vi "0520_Controle_servo_braço.vi"() -> ()   [LabVIEW 2017]
uses:
  <vilib>/Utility/error.llb/Error Cluster From Error Code.vi
  <vilib>/myRIO/Common/Instrument Driver Framework/myRIO v1.0/PWM/vis/myRIO v1.0 Write PWM.vi
  <vilib>/myRIO/Instrument Drivers/Onboard IO/PWM/PWM.lvlib
panel:
  in  "Numeric":dbl
  in  "Record Button":bool
  in  "Play Button":bool
  in  "Array":dbl[][](array[numeric])
  in  "Comprimento de pulso R7":dbl(knob)=1.5 step=0.05 scale=0.25..0.125
  out "error out 7":errorcluster
  out "error out 6":errorcluster
  out "error out 5":errorcluster
  out "error out 4":errorcluster
  out "error out 3":errorcluster
  in  "error in (no error) 7":errorcluster
  in  "error in (no error) 6":errorcluster
  in  "error in (no error) 5":errorcluster
  in  "error in (no error) 4":errorcluster
  in  "error in (no error) 3":errorcluster
  in  "Comprimento de pulso R6":dbl(knob)=90.0 min=90.0 max=300.0 step=3.0 scale=90.0..300.0
  in  "Comprimento de pulso R5":dbl(knob)=0.125 min=0.0 max=180.0 step=3.0 scale=0.0..180.0
  in  "Comprimento de pulso R4":dbl(knob) min=-180.0 max=0.0 step=3.0
  in  "Comprimento de pulso R3":dbl(knob)=0.125 min=0.025 max=0.125 step=0.001 scale=0.025..0.125
  in  "Comprimento de pulso R2":dbl(knob)=0.125 min=-90.0 max=90.0 step=1.0 scale=-90.0..90.0
  out "error out 2":errorcluster
  in  "error in (no error) 2":errorcluster
  out "error out":errorcluster
  in  "error in (no error)":errorcluster
  in  "Comprimento de pulso R1":dbl(knob)=0.125 min=0.025 max=0.125 step=0.001 scale=0.025..0.125
  in  "Stop Button":bool
  # "Range: 0,025 - 0,125\n\n3° = 0,00125\n\nLink 1 - (0,00125/3)x + 0,1\n0,125 -> 60°\n0,1 -> 0°\n0,0625 -> -90\n0,025 -> -180°\n\nLink 2 - -(0,00125/3)x + 0,1\n0,025 -> 180°\n0,0625 -> 90°\n0,1 -> 0°\n0,125 -> -60°\n\nLink 3 - (0,00125/3)x - 0,0125\n0,125 -> 300°\n0,105 -> 270° \n0,63 -> 180°\n0,025 -> 90°\n\n9° = 0,05\n\nLink 5 - (0,005/9)x + 0,075\n0,125 -> 90°\n0,075 -> 0°\n0,025 ->-90°"
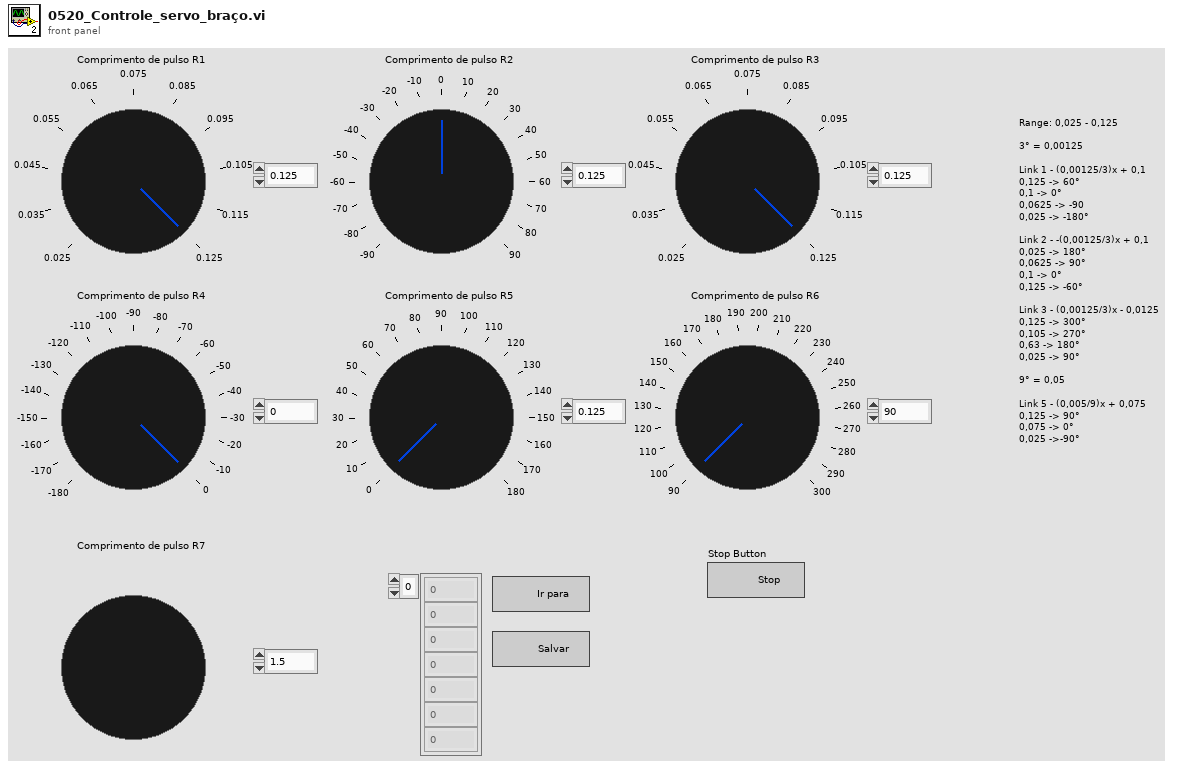
[diagram p1: front panel]
types:
  T1 = typedef "PWM.lvlib/PWM Reference.ctl" = cluster{"myRIO Reference":T2, "PWM Channels Enum":T6, "PWM Configuration":T7}
  T2 = typedef "myRIO Generic Hardware Reference.ctl" = cluster{"myRIO Model":T3, "myRIO Hardware Reference":T4}
  T3 = typedef "Hardware Version Enum.ctl" = enum16{"Unknown", "myRIO-1900", "myRIO-1950", "roboRIO", "NI ELVIS RIO CM"}
  T4 = typedef "myRIO v1.0 Reference.ctl" = cluster{"Generic FPGA Reference":T5, "Allow multiple opens":bool}
  T5 = typedef "Generic FPGA Reference.ctl" = refnum<k20>
  T6 = typedef "PWM Channels Enum.ctl" = enum16{"Not Connected", "C/PWM0", "C/PWM1", "A/PWM0", "A/PWM1", "A/PWM2", "B/PWM0", "B/PWM1", "B/PWM2", "PWM/PWM0", "PWM/PWM1", "PWM/PWM2", "PWM/PWM3", "PWM/PWM4", "PWM/PWM5", "PWM/PWM6", "PWM/PWM7", "PWM/PWM8", "PWM/PWM9"}
  T7 = typedef "PWM.lvlib/PWM Configuration.ctl" = cluster{"Frequency":dbl, "Duty Cycle":dbl}
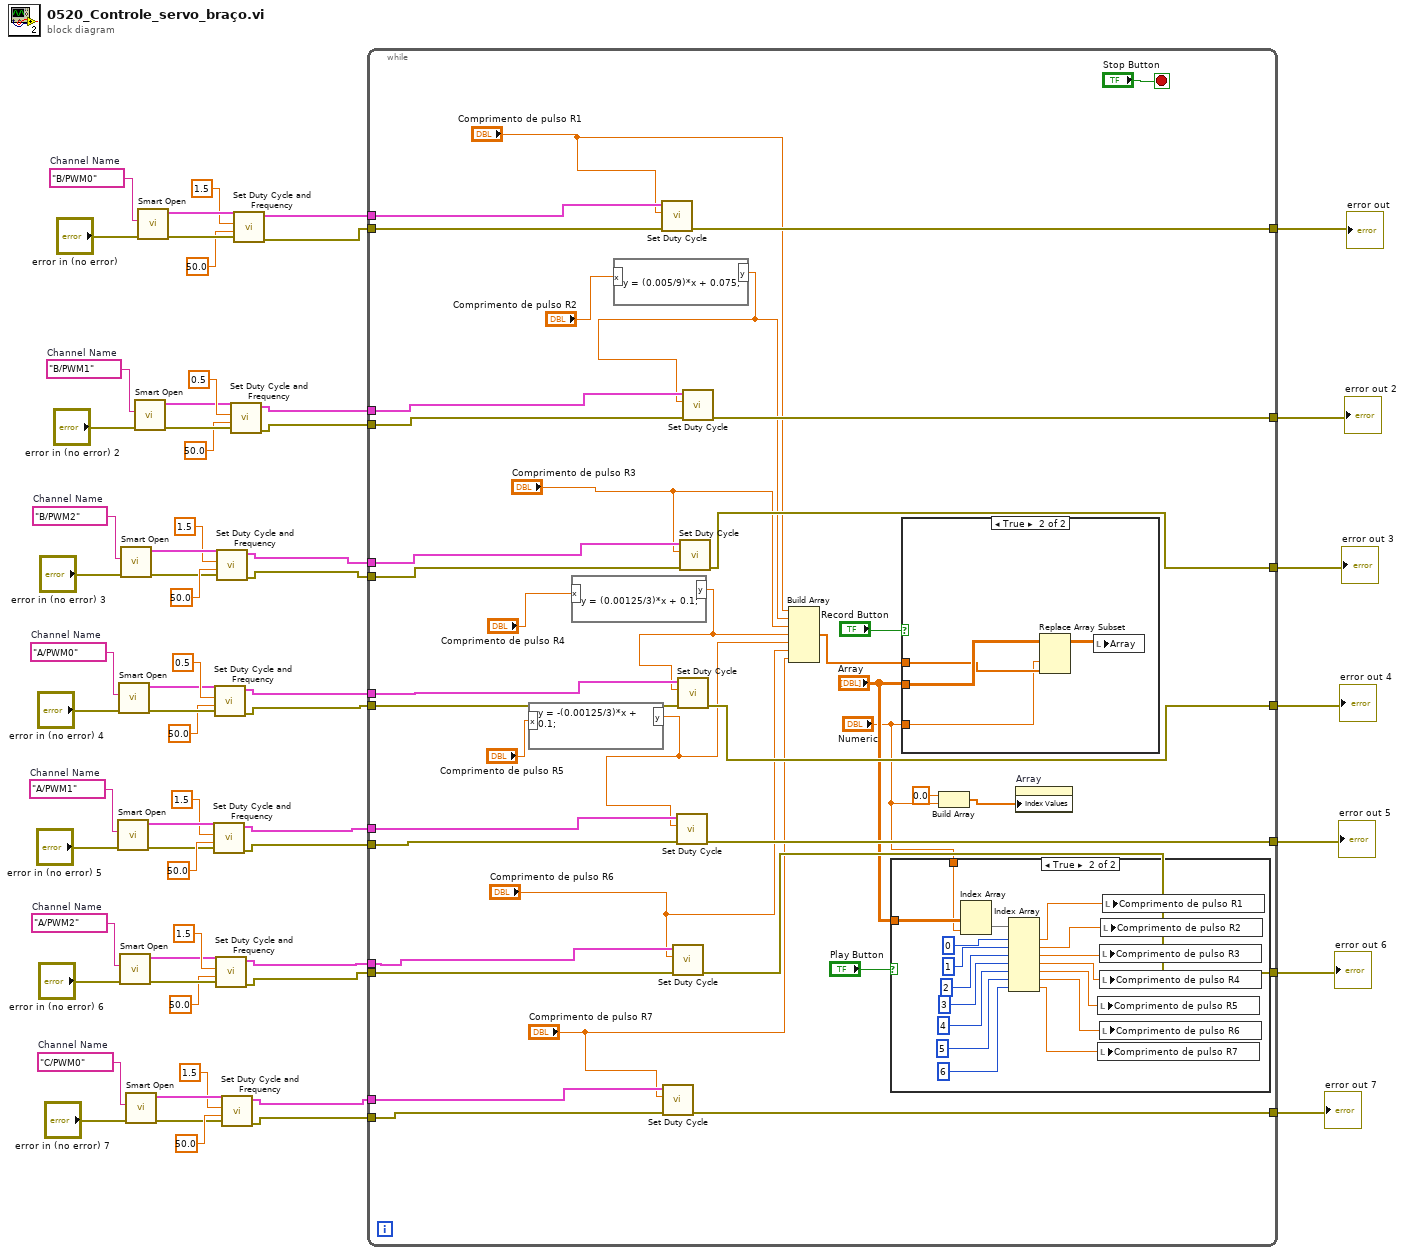
[diagram p0: block diagram]
diagram:
  w19 = tag "C/PWM0"  # Channel Name
  w24 = tag "A/PWM2"  # Channel Name
  w31 = tag "A/PWM1"  # Channel Name
  w36 = tag "A/PWM0"  # Channel Name
  w43 = tag "B/PWM2"  # Channel Name
  w52 = tag "B/PWM1"  # Channel Name
  w62 = tag "B/PWM0"  # Channel Name
  n1 = call <vilib>:"Smart Open.vi"("error in (no error)"="error in (no error) 5", "Channel Name"=w31) -> ("error out"=w30:errorcluster, "PWM Ref Out"=w29:T1)  [unwired: 8 in]
  n2 = call <vilib>:"Smart Open.vi"("error in (no error)"="error in (no error) 4", "Channel Name"=w36) -> ("error out"=w37:errorcluster, "PWM Ref Out"=w38:T1)  [unwired: 8 in]
  n3 = call <vilib>:"Smart Open.vi"("error in (no error)"="error in (no error) 6", "Channel Name"=w24) -> ("error out"=w25:errorcluster, "PWM Ref Out"=w26:T1)  [unwired: 8 in]
  n4 = call <vilib>:"Smart Open.vi"("error in (no error)"="error in (no error) 3", "Channel Name"=w43) -> ("error out"=w42:errorcluster, "PWM Ref Out"=w41:T1)  [unwired: 8 in]
  n5 = call <vilib>:"Smart Open.vi"("error in (no error)"="error in (no error) 7", "Channel Name"=w19) -> ("error out"=w18:errorcluster, "PWM Ref Out"=w17:T1)  [unwired: 8 in]
  n6 = call <vilib>:"Smart Open.vi"("error in (no error)"="error in (no error) 2", "Channel Name"=w52) -> ("error out"=w53:errorcluster, "PWM Ref Out"=w54:T1)  [unwired: 8 in]
  n7 = call <vilib>:"Smart Open.vi"("error in (no error)"="error in (no error)", "Channel Name"=w62) -> ("error out"=w61:errorcluster, "PWM Ref Out"=w60:T1)  [unwired: 8 in]
  n8 = call <vilib>:"Set Duty Cycle and Frequency.vi"("error in (no error)"=w30, "Frequency [Hz]"=50.0, "Duty Cycle"=1.5, "PWM Ref In"=w29) -> ("error out"=w6:errorcluster, "PWM Ref Out"=w5:T1)  [unwired: 5 in]
  n9 = call <vilib>:"Set Duty Cycle and Frequency.vi"("error in (no error)"=w37, "Frequency [Hz]"=50.0, "Duty Cycle"=0.5, "PWM Ref In"=w38) -> ("error out"=w4:errorcluster, "PWM Ref Out"=w3:T1)  [unwired: 5 in]
  n10 = call <vilib>:"Set Duty Cycle and Frequency.vi"("error in (no error)"=w25, "Frequency [Hz]"=50.0, "Duty Cycle"=1.5, "PWM Ref In"=w26) -> ("error out"=w8:errorcluster, "PWM Ref Out"=w7:T1)  [unwired: 5 in]
  n11 = call <vilib>:"Set Duty Cycle and Frequency.vi"("error in (no error)"=w42, "Frequency [Hz]"=50.0, "Duty Cycle"=1.5, "PWM Ref In"=w41) -> ("error out"=w2:errorcluster, "PWM Ref Out"=w1:T1)  [unwired: 5 in]
  n12 = call <vilib>:"Set Duty Cycle and Frequency.vi"("error in (no error)"=w18, "Frequency [Hz]"=50.0, "Duty Cycle"=1.5, "PWM Ref In"=w17) -> ("error out"=w9:errorcluster, "PWM Ref Out"=w10:T1)  [unwired: 5 in]
  n13 = call <vilib>:"Set Duty Cycle and Frequency.vi"("error in (no error)"=w53, "Frequency [Hz]"=50.0, "Duty Cycle"=0.5, "PWM Ref In"=w54) -> ("error out"=w49:errorcluster, "PWM Ref Out"=w50:T1)  [unwired: 5 in]
  n14 = call <vilib>:"Set Duty Cycle and Frequency.vi"("error in (no error)"=w61, "Frequency [Hz]"=50.0, "Duty Cycle"=1.5, "PWM Ref In"=w60) -> ("error out"=w58:errorcluster, "PWM Ref Out"=w59:T1)  [unwired: 5 in]
  n15 = while {
    tunnel: w59 -> [w101]
    tunnel: w58 -> [w100]
    tunnel: [w99] -> w57
    tunnel: w50 -> [w98]
    tunnel: w49 -> [w97]
    tunnel: [w96] -> w48
    tunnel: [w95] -> w15
    tunnel: [w94] -> w14
    tunnel: [w93] -> w13
    tunnel: [w92] -> w12
    tunnel: [w91] -> w11
    tunnel: w10 -> [w90]
    tunnel: w9 -> [w89]
    tunnel: w8 -> [w88]
    tunnel: w7 -> [w87]
    tunnel: w6 -> [w86]
    tunnel: w5 -> [w85]
    tunnel: w4 -> [w84]
    tunnel: w3 -> [w83]
    tunnel: w2 -> [w82]
    tunnel: w1 -> [w81]
    stop <- "Stop Button" stop-if-true
    n16 = formula code="y = -(0.00125/3)*x + 0.1;"("x"="Comprimento de pulso R5") -> ("y"=w68:dbl)
    n17 = formula code="y = (0.00125/3)*x + 0.1;"("x"="Comprimento de pulso R4") -> ("y"=w69:dbl)
    n18 = formula code="y = (0.005/9)*x + 0.075;"("x"="Comprimento de pulso R2") -> ("y"=w65:dbl)
    n19 = call <vilib>:"Set Duty Cycle.vi"("error in (no error)"=w100, "Duty Cycle"="Comprimento de pulso R1", "PWM Ref In"=w101) -> ("error out"=w99:errorcluster)  [unwired: 6 in, 1 out]
    n20 = call <vilib>:"Set Duty Cycle.vi"("error in (no error)"=w89, "Duty Cycle"="Comprimento de pulso R7", "PWM Ref In"=w90) -> ("error out"=w91:errorcluster)  [unwired: 6 in, 1 out]
    n21 = call <vilib>:"Set Duty Cycle.vi"("error in (no error)"=w88, "Duty Cycle"="Comprimento de pulso R6", "PWM Ref In"=w87) -> ("error out"=w92:errorcluster)  [unwired: 6 in, 1 out]
    n22 = call <vilib>:"Set Duty Cycle.vi"("error in (no error)"=w86, "Duty Cycle"=w68, "PWM Ref In"=w85) -> ("error out"=w93:errorcluster)  [unwired: 6 in, 1 out]
    n23 = call <vilib>:"Set Duty Cycle.vi"("error in (no error)"=w84, "Duty Cycle"=w69, "PWM Ref In"=w83) -> ("error out"=w94:errorcluster)  [unwired: 6 in, 1 out]
    n24 = call <vilib>:"Set Duty Cycle.vi"("error in (no error)"=w82, "Duty Cycle"="Comprimento de pulso R3", "PWM Ref In"=w81) -> ("error out"=w95:errorcluster)  [unwired: 6 in, 1 out]
    n25 = call <vilib>:"Set Duty Cycle.vi"("error in (no error)"=w97, "Duty Cycle"=w65, "PWM Ref In"=w98) -> ("error out"=w96:errorcluster)  [unwired: 6 in, 1 out]
    n26 = Build Array("Comprimento de pulso R1", w65, "Comprimento de pulso R3", w69, w68, "Comprimento de pulso R6", "Comprimento de pulso R7") -> (w79:dbl[])
    n27 = case shown="True" "Play Button" {
      tunnel: "Array" -> [_ w119]
      tunnel: "Numeric" -> [_ w118]
      frame False {
      }
      frame True {
        n28 = Index Array(array=w119, index (col)=w118) -> (element=w117:dbl[])  [unwired: 1 in]
        n29 = Index Array(array=w117, index #1=0 ("index"), index #2=1 ("index"), index #3=2 ("index"), index #4=3 ("index"), index #5=4 ("index"), index #6=5 ("index"), index #7=6 ("index")) -> (element #1=w109:dbl, element #2=w108:dbl, element #3=w107:dbl, element #4=w106:dbl, element #5=w105:dbl, element #6=w104:dbl, element #7=w103:dbl)
        n30 = local write "Comprimento de pulso R5"(w105) -> ()
        n31 = local write "Comprimento de pulso R7"(w103) -> ()
        n32 = local write "Comprimento de pulso R3"(w107) -> ()
        n33 = local write "Comprimento de pulso R4"(w106) -> ()
        n34 = local write "Comprimento de pulso R6"(w104) -> ()
        n35 = local write "Comprimento de pulso R2"(w108) -> ()
        n36 = local write "Comprimento de pulso R1"(w109) -> ()
      }
    }
    n37 = case shown="True" "Record Button" {
      tunnel: "Array" -> [_ w123]
      tunnel: w79 -> [_ w121]
      tunnel: "Numeric" -> [_ w120]
      frame False {
      }
      frame True {
        n38 = Replace Array Subset(array=w123, new element=w121, index (col)=w120) -> (w122:dbl[][])  [unwired: 1 in]
        n39 = local write "Array"(w122) -> ()
      }
    }
    n40 = Build Array(0.0 ("element"), "Numeric") -> (w77:dbl[])
    n41 = property on="Array" class="Arr (strict)"("Index Values"=w77) -> ()  [unwired: 2 in, 2 out]
  }
  "error out" <- w57
  "error out 2" <- w48
  "error out 3" <- w15
  "error out 4" <- w14
  "error out 5" <- w13
  "error out 6" <- w12
  "error out 7" <- w11
